vi "act-0010-1-cor.vi"() -> ()   [LabVIEW 2010]
uses:
  lv_01/lv_01.lvlib
panel:
  out "affichage":dbl caption="Temp simulée en °F"
  in  "sélecteur":bool
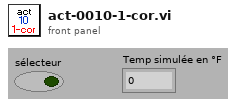
[diagram p1: front panel]
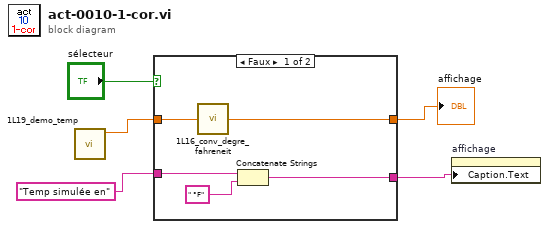
[diagram p0: block diagram]
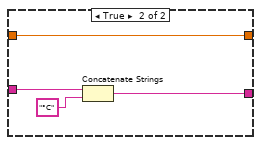
[diagram p2: hidden frame]
diagram:
  n1 = call "1L19_demo_temp.vi"() -> ("temp"=w4:dbl)  [unwired: 6 in, 1 out]
  n2 = case shown="Faux" "sélecteur" {
    tunnel: w4 -> [w10 w12]
    tunnel: "Temp simulée en" -> [w9 w13]
    tunnel: [w7 w11] -> w1
    tunnel: [w6 w12] -> w2
    frame False {
      n3 = call "1L16_conv_degre_fahreneit.vi"("Deg C"=w10) -> ("Deg F"=w6:dbl)
      n4 = Concatenate Strings(w9, " °F" ("Étiquette.Texte")) -> (w7:string)
    }
    frame True {
      n5 = Concatenate Strings(w13, "°C" ("Étiquette.Texte")) -> (w11:string)
    }
  }
  "affichage" <- w2
  n6 = property on="affichage" class="NumDig (strict)"("Caption.Text"=w1) -> ()  [unwired: 2 in, 2 out]
